vi "Meas Result Add Reading.vi"(4 "reading":T2={"U [V]"=nan, "f [Hz]"=nan, "unc(U) [V] (k=2)"=nan, "formated rdg str"=""}, 5 "thermo":T1, 6 "reading per phase":T3[](array[typedef]), 7 "fid count (default: 1)":i32=1, 8 "error in":errorcluster, 9 "f [Hz]":dbl, 10 "freq. id (default: 0)":i32, 11 "results ref":refnum<vi>) -> (0 "error out":errorcluster, 3 "result data":T6)   [LabVIEW 2020]
doc: "Adds single reading (per each phase) to the result."
uses:
  Meas Results.ctl
  bridge/Bridge Frequency Readings Data.ctl
  drivers/TWM client/Meas Proc QWTB Spectrum Data.ctl
  drivers/TWM client/TWM Phase Info.ctl
  bridge/Bridge Reading Data.ctl
  dvm/dvm Reading.ctl
  thermo/thermo_read.ctl
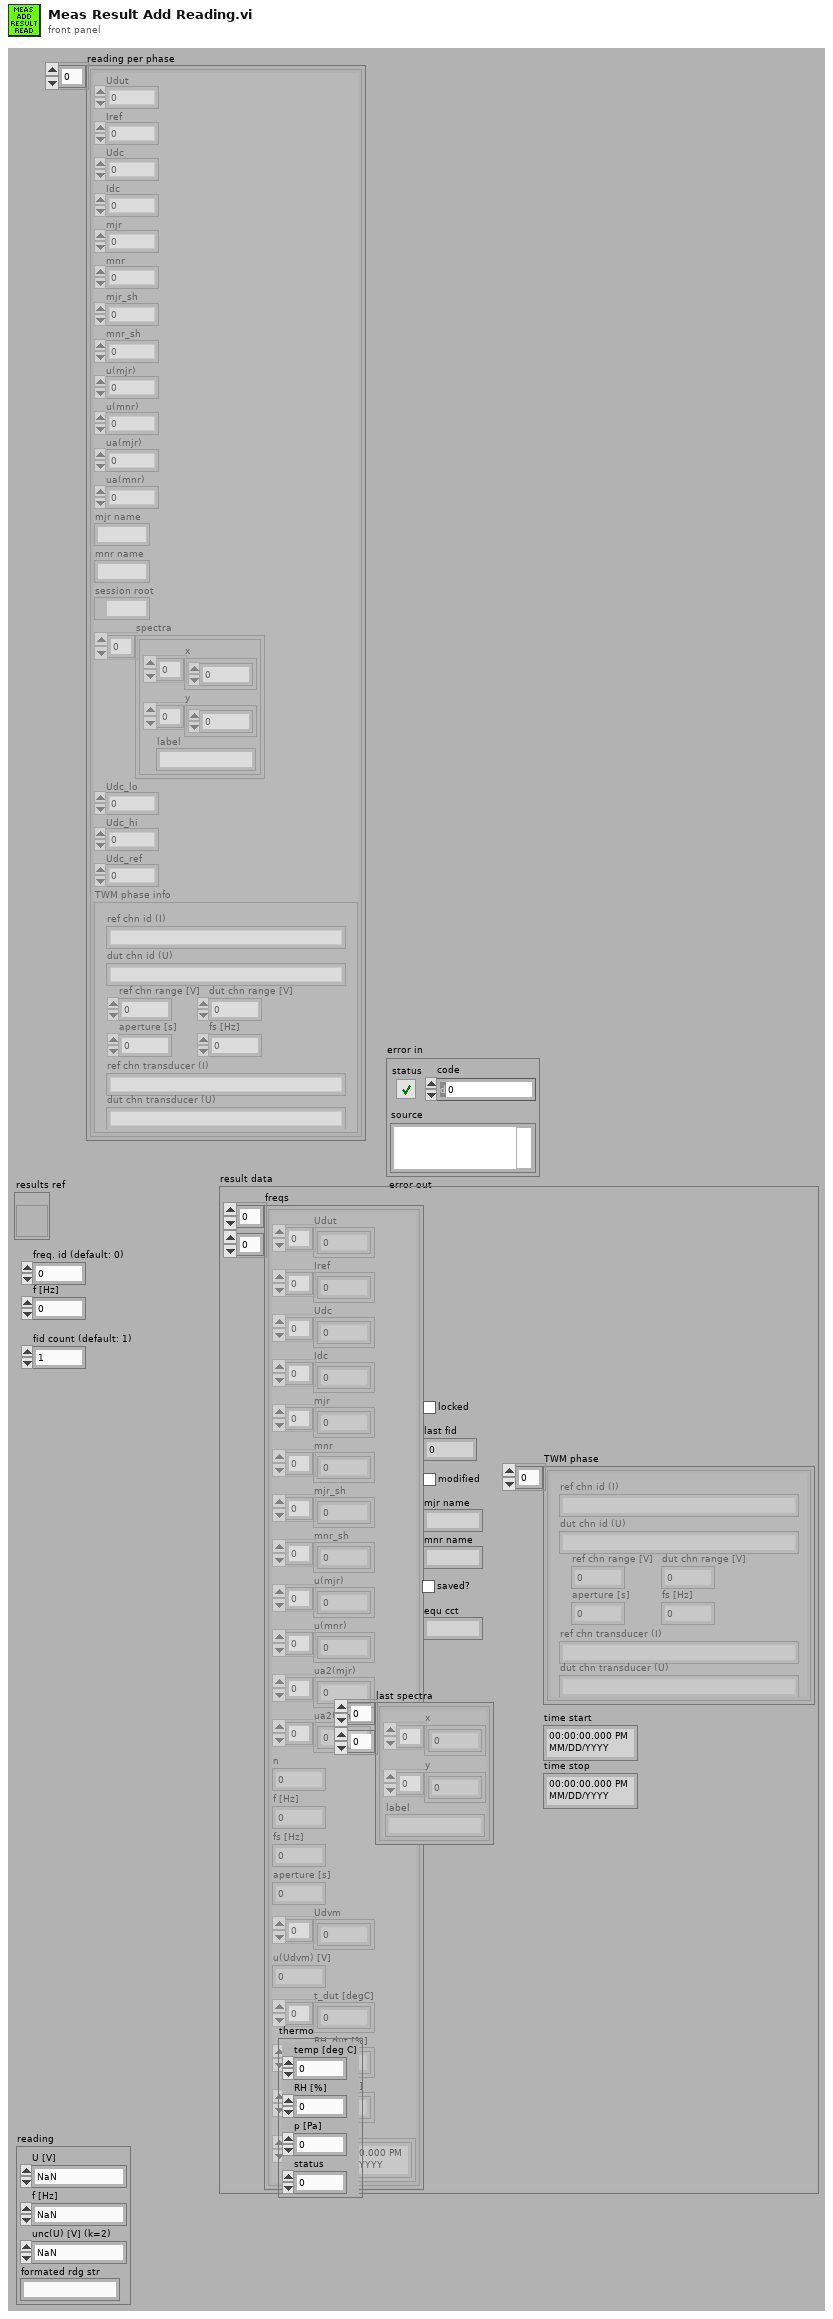
[diagram p1: front panel]
types:
  T1 = typedef "thermo_read.ctl" = cluster{"temp [deg C]":dbl, "RH [%]":dbl, "p [Pa]":dbl, "status":i32}
  T2 = typedef "dvm Reading.ctl" = cluster{"U [V]":dbl, "f [Hz]":dbl, "unc(U) [V] (k=2)":dbl, "formated rdg str":string}
  T3 = typedef "Bridge Reading Data.ctl" = cluster{"Udut":dbl, "Iref":dbl, "Udc":dbl, "Idc":dbl, "mjr":dbl, "mnr":dbl, "mjr_sh":dbl, "mnr_sh":dbl, "u(mjr)":dbl, "u(mnr)":dbl, "ua(mjr)":dbl, "ua(mnr)":dbl, "mjr name":string, "mnr name":string, "session root":path, "spectra":T4[], "Udc_lo":dbl, "Udc_hi":dbl, "Udc_ref":dbl, "TWM phase info":T5}
  T4 = typedef "Meas Proc QWTB Spectrum Data.ctl" = cluster{"x":sgl[], "y":sgl[], "label":string}
  T5 = typedef "TWM Phase Info.ctl" = cluster{"ref chn id (I)":string, "dut chn id (U)":string, "ref chn range [V]":dbl, "dut chn range [V]":dbl, "aperture [s]":dbl, "fs [Hz]":dbl, "ref chn transducer (I)":string, "dut chn transducer (U)":string}
  T6 = typedef "Meas Results.ctl" = cluster{"freqs":T7[][], "locked":bool, "last fid":i32, "modified":bool, "mjr name":string, "mnr name":string, "last spectra":T4[][], "saved?":bool, "TWM phase":T5[], "time start":timestamp, "time stop":timestamp, "equ cct":string}
  T7 = typedef "Bridge Frequency Readings Data.ctl" = cluster{"Udut":dbl[], "Iref":dbl[], "Udc":dbl[], "Idc":dbl[], "mjr":dbl[], "mnr":dbl[], "mjr_sh":dbl[], "mnr_sh":dbl[], "u(mjr)":dbl[], "u(mnr)":dbl[], "ua2(mjr)":dbl[], "ua2(mnr)":dbl[], "n":i32, "f [Hz]":dbl, "fs [Hz]":dbl, "aperture [s]":dbl, "Udvm":dbl[], "u(Udvm) [V]":dbl, "t_dut [degC]":dbl[], "RH_dut [%]":dbl[], "p_dut [Pa]":dbl[], "timestamp":timestamp[]}
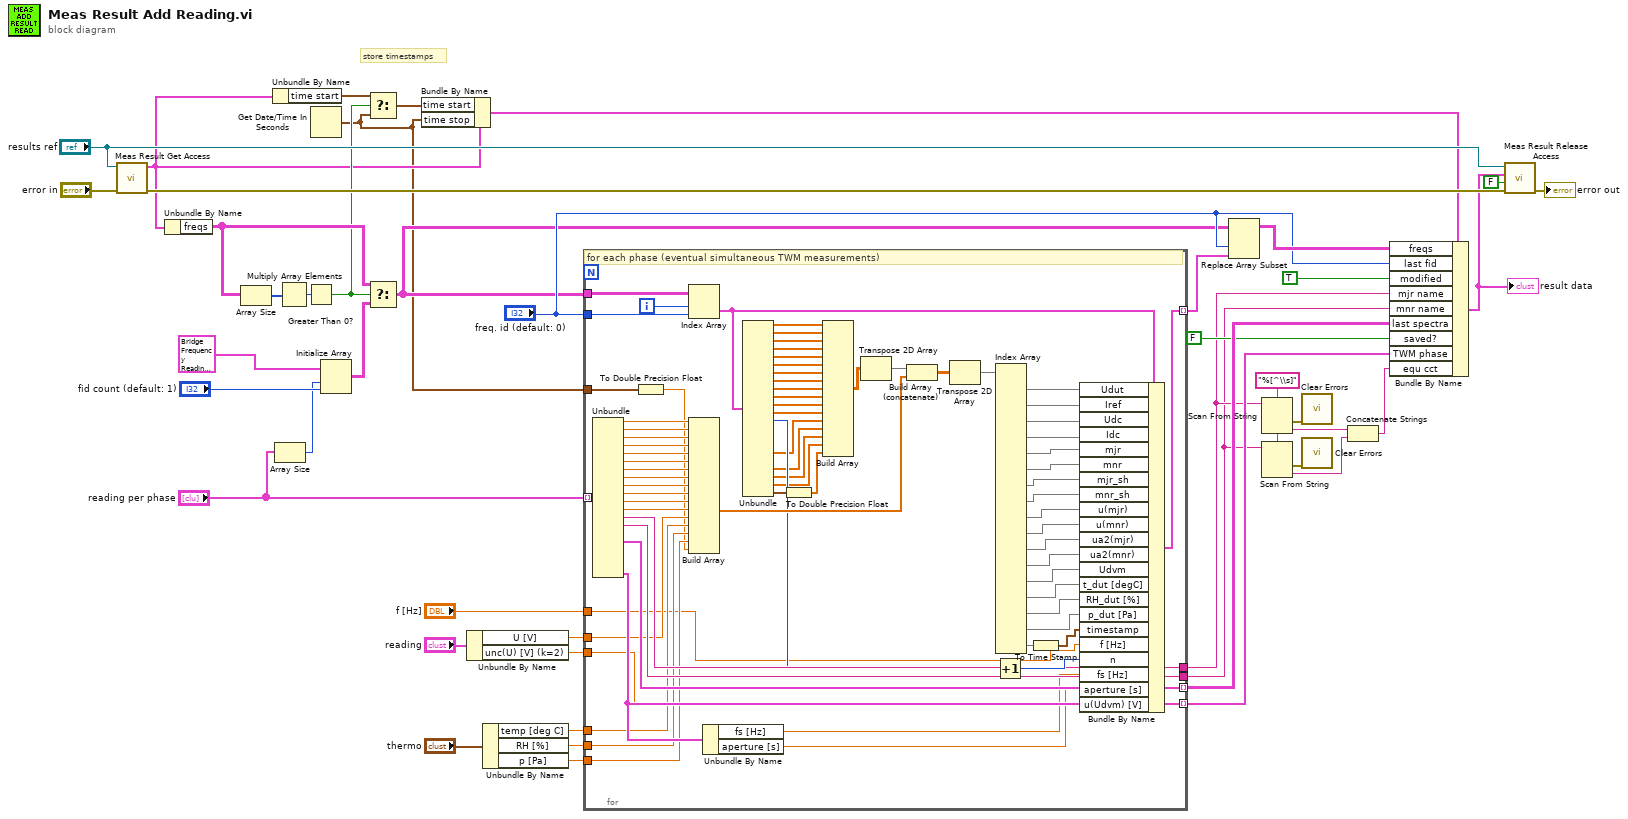
[diagram p0: block diagram]
diagram:
  w13 = "%[^\\s]" ("format string")
  # "store timestamps"
  n1 = call "Meas Result Get Access.vi"("error in"="error in", "results ref"="results ref") -> ("error out"=w44:errorcluster, "results data"=w19:T6)  [unwired: 8 in]
  n2 = Unbundle By Name(w19) -> ("freqs"=w31:T7[][])
  n3 = Array Size(array=w31) -> (size(s)=w34:i32[])
  n4 = Unbundle By Name(w19) -> ("time start"=w20:timestamp)
  n5 = Array Size(array="reading per phase") -> (size(s)=w24:i32)
  n6 = Multiply Array Elements(1:w34) -> (0:w35:i32)
  n7 = Greater Than 0?(x=w35) -> (x > 0?=w21:bool)
  n8 = Get Date/Time In Seconds() -> (seconds since 1Jan1904=w1:timestamp)
  n9 = Initialize Array(T7 {"Udut"=[], "Iref"=[], "Udc"=[], "Idc"=[], "mjr"=[], "mnr"=[], "mjr_sh"=[], "mnr_sh"=[], "u(mjr)"=[], "u(mnr)"=[], "ua2(mjr)"=[], "ua2(mnr)"=[], "n"=0, "f [Hz]"=0.0, "fs [Hz]"=0.0, "aperture [s]"=0.0, "Udvm"=[], "u(Udvm) [V]"=0.0, "t_dut [degC]"=[], "RH_dut [%]"=[], "p_dut [Pa]"=[], "timestamp"=[]} ("output cluster"), w24, "fid count (default: 1)") -> (w32:T7[][])
  n10 = Select(t=w20, s=w21, f=w1) -> (s? t:f=w17:timestamp)
  n11 = Select(t=w31, s=w21, f=w32) -> (s? t:f=w27:T7[][])
  n12 = Bundle By Name(cluster=w19, "time start"=w17, "time stop"=w1) -> (w18:T6)
  n13 = Unbundle By Name("reading") -> ("U [V]"=w14:dbl, "unc(U) [V] (k=2)"=w15:dbl)
  n14 = Unbundle By Name("thermo") -> ("temp [deg C]"=w4:dbl, "RH [%]"=w3:dbl, "p [Pa]"=w2:dbl)
  n15 = for {
    tunnel: [w104] -> w30 mode=indexing
    tunnel: w27 -> [w103]
    tunnel: "f [Hz]" -> [w54]
    tunnel: "reading per phase" -> [w100] mode=indexing
    tunnel: [w88] -> w10
    tunnel: [w87] -> w9
    tunnel: [w71] -> w36 mode=indexing
    tunnel: "freq. id (default: 0)" -> [w70]
    tunnel: [w67] -> w22 mode=indexing
    tunnel: w15 -> [w64]
    tunnel: w14 -> [w61]
    tunnel: w4 -> [w60]
    tunnel: w3 -> [w59]
    tunnel: w2 -> [w58]
    tunnel: w1 -> [w46]
    i -> [w69]
    # "for each phase (eventual simultaneous TWM measurements)"
    n16 = Unbundle(w100) -> ("Udut"=w99:dbl, "Iref"=w98:dbl, "Udc"=w97:dbl, "Idc"=w96:dbl, "mjr"=w95:dbl, "mnr"=w94:dbl, "mjr_sh"=w77:dbl, "mnr_sh"=w76:dbl, "u(mjr)"=w75:dbl, "u(mnr)"=w74:dbl, "ua(mjr)"=w73:dbl, "ua(mnr)"=w72:dbl, "mjr name"=w88:string, "mnr name"=w87:string, "spectra"=w71:T4[], "TWM phase info"=w67:T5)  [unwired: 4 out]
    n17 = To Double Precision Float(number=w46) -> (double precision float=w45:dbl)
    n18 = Index Array(array=w103, index (row)=w69, index (col)=w70) -> (element=w68:T7)
    n19 = Build Array(w99, w98, w97, w96, w95, w94, w77, w76, w75, w74, w73, w72, w61, w60, w59, w58, w45) -> (w93:dbl[])
    n20 = Unbundle By Name(w67) -> ("fs [Hz]"=w66:dbl, "aperture [s]"=w65:dbl)
    n21 = Unbundle(w68) -> ("Udut"=w119:dbl[], "Iref"=w118:dbl[], "Udc"=w117:dbl[], "Idc"=w116:dbl[], "mjr"=w115:dbl[], "mnr"=w114:dbl[], "mjr_sh"=w92:dbl[], "mnr_sh"=w91:dbl[], "u(mjr)"=w90:dbl[], "u(mnr)"=w89:dbl[], "ua2(mjr)"=w79:dbl[], "ua2(mnr)"=w78:dbl[], "n"=w80:i32, "Udvm"=w63:dbl[], "t_dut [degC]"=w53:dbl[], "RH_dut [%]"=w52:dbl[], "p_dut [Pa]"=w51:dbl[], "timestamp"=w50:timestamp[])  [unwired: 4 out]
    n22 = To Double Precision Float(number=w50) -> (double precision float=w49:dbl[])
    n23 = Build Array(w119, w118, w117, w116, w115, w114, w92, w91, w90, w89, w79, w78, w63, w53, w52, w51, w49) -> (w113:dbl[][])
    n24 = Transpose 2D Array(2D array=w113) -> (transposed array=w102:dbl[][])
    n25 = Build Array (concatenate)(w102, w93) -> (w112:dbl[][])
    n26 = Transpose 2D Array(2D array=w112) -> (transposed array=w101:dbl[][])
    n27 = Increment(x=w80) -> (x+1=w105:i32)
    n28 = Index Array(array=w101) -> (element #1=w111:dbl[], element #2=w110:dbl[], element #3=w109:dbl[], element #4=w108:dbl[], element #5=w107:dbl[], element #6=w106:dbl[], element #7=w81:dbl[], element #8=w82:dbl[], element #9=w83:dbl[], element #10=w84:dbl[], element #11=w85:dbl[], element #12=w86:dbl[], element #13=w62:dbl[], element #14=w57:dbl[], element #15=w56:dbl[], element #16=w55:dbl[], element #17=w48:dbl[])  [unwired: 34 in]
    n29 = To Time Stamp(1:w48) -> (0:w47:timestamp[])
    n30 = Bundle By Name(cluster=w68, "Udut"=w111, "Iref"=w110, "Udc"=w109, "Idc"=w108, "mjr"=w107, "mnr"=w106, "mjr_sh"=w81, "mnr_sh"=w82, "u(mjr)"=w83, "u(mnr)"=w84, "ua2(mjr)"=w85, "ua2(mnr)"=w86, "Udvm"=w62, "t_dut [degC]"=w57, "RH_dut [%]"=w56, "p_dut [Pa]"=w55, "timestamp"=w47, "f [Hz]"=w54, "n"=w105, "fs [Hz]"=w66, "aperture [s]"=w65, "u(Udvm) [V]"=w64) -> (w104:T7)
  }
  n31 = Replace Array Subset(array=w27, new element=w30, index (col)="freq. id (default: 0)") -> (w29:T7[][])  [unwired: 1 in]
  n32 = Scan From String(format string=w13, input string=w10) -> (error out=w12:errorcluster, output 1=w8:string)  [unwired: 3 in, 2 out]
  n33 = Scan From String(format string=w13, input string=w9) -> (error out=w11:errorcluster, output 1=w7:string)  [unwired: 3 in, 2 out]
  n34 = call <vilib>:"Clear Errors.vi"("error in (no error)"=w12) -> ()  [unwired: 5 in, 2 out]
  n35 = call <vilib>:"Clear Errors.vi"("error in (no error)"=w11) -> ()  [unwired: 5 in, 2 out]
  n36 = Concatenate Strings(w8, w7) -> (w6:string)
  n37 = Bundle By Name(cluster=w18, "freqs"=w29, "last fid"="freq. id (default: 0)", "modified"=TRUE, "mjr name"=w10, "mnr name"=w9, "last spectra"=w36, "saved?"=FALSE, "TWM phase"=w22, "equ cct"=w6) -> (w43:T6)
  "result data" <- w43
  n38 = call "Meas Result Release Access.vi"("error in"=w44, "Release only (True)"=FALSE, "results data in"=w43, "results ref"="results ref") -> ("error out"=→"error out":errorcluster)  [unwired: 7 in]
